vi "Wait Interval.vi"(9 "Channel":i16, 10 "Interval unit":enum16{"ms", "s", "min"}(ring), 11 "Interval":u32=9) -> (3 "Wait":u32)   [LabVIEW 2015]
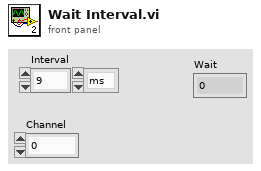
[diagram p1: front panel]
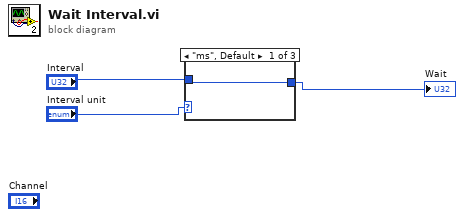
[diagram p0: block diagram]
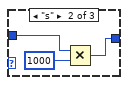
[diagram p2: hidden frame]
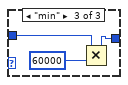
[diagram p3: hidden frame]
diagram:
  n1 = case shown="\"ms\", Default" "Interval unit" {
    tunnel: [w4 w7 w10] -> w1
    tunnel: "Interval" -> [w4 w5 w8]
    frame "ms", Default {
    }
    frame "s" {
      n2 = Multiply(x=w5, y=u32 1000) -> (x*y=w7:u32)
    }
    frame "min" {
      n3 = Multiply(x=w8, y=u32 60000) -> (x*y=w10:u32)
    }
  }
  "Wait" <- w1
